vi "GlobalGetSetMeasurementType.vi"() -> ()   [LabVIEW 2011]
panel:
  in  "Measurement-Type":enum32{"Diffusion", "Imaging"}(ring)
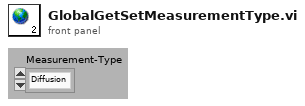
[diagram p1: front panel]
diagram:
